vi "Manipulator Set Approach.vi"(8 "error in (no error)":errorcluster, 10 "SET/RESET":bool, 11 "VISA resource in":refnum<visa-resource-name>="COM1") -> (0 "error out":errorcluster, 2 "Response":string, 3 "VISA resource out":refnum<visa-resource-name>)   [LabVIEW 2012, in "Scientifica Manipulator Daemon.lvlib"]
uses:
  Scientifica Manipulator Daemon.lvlib
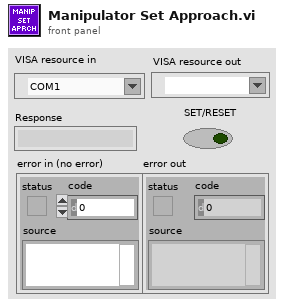
[diagram p1: front panel]
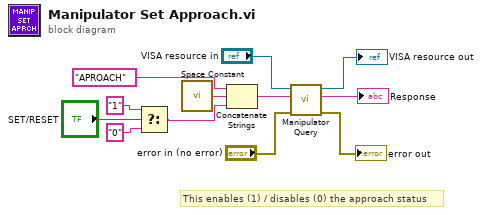
[diagram p0: block diagram]
diagram:
  # "This enables (1) / disables (0) the approach status"
  n1 = Select(t="1", s="SET/RESET", f="0") -> (s? t:f=w1:string)
  n2 = call <vilib>:"Space Constant.vi"() -> ("String"=w7:string)
  n3 = Concatenate Strings("APROACH", w7, w1) -> (w6:string)
  n4 = call "Manipulator Query.vi"("error in (no error)"="error in (no error)", "Command"=w6, "VISA resource in"="VISA resource in") -> ("error out"=→"error out":errorcluster, "Response"=→"Response":string, "VISA resource out"=→"VISA resource out":refnum<visa-resource-name>)  [unwired: 5 in, 1 out]
